vi "GET Async.vi"(0 "client handle":T1, 1 "output file":path=path "", 5 "url":string, 11 "error in (no error)":errorcluster, 12 "timeout (10000)":i32=10000) -> (4 "client handle out":T1, 6 "get async handle":T2, 10 "headers":string, 15 "error out":errorcluster)   [LabVIEW 2019, in "HTTP Client Extensions.lvlib" / "Get Async.lvlib"]
uses:
  Get Async.lvlib
  <vilib>/httpClient/ClientHandle.ctl
  controls/Refnum Type.ctl
  controls/Refnum Type - Enum.ctl
  HTTP GET Async/GET Async.lvclass
  <vilib>/httpClient/LabVIEWHTTPClient.lvlib
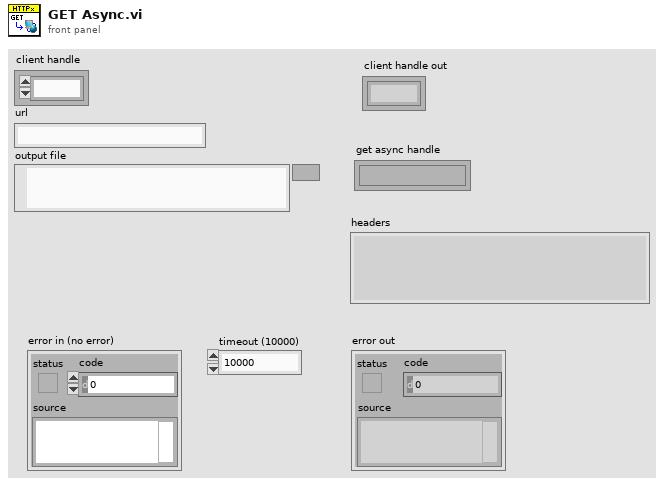
[diagram p1: front panel]
types:
  T1 = typedef "LabVIEWHTTPClient.lvlib/ClientHandle.ctl" = refnum<k1>
  T2 = typedef "HTTP Client Extensions.lvlib/Get Async.lvlib/Refnum Type.ctl" = refnum<k1>
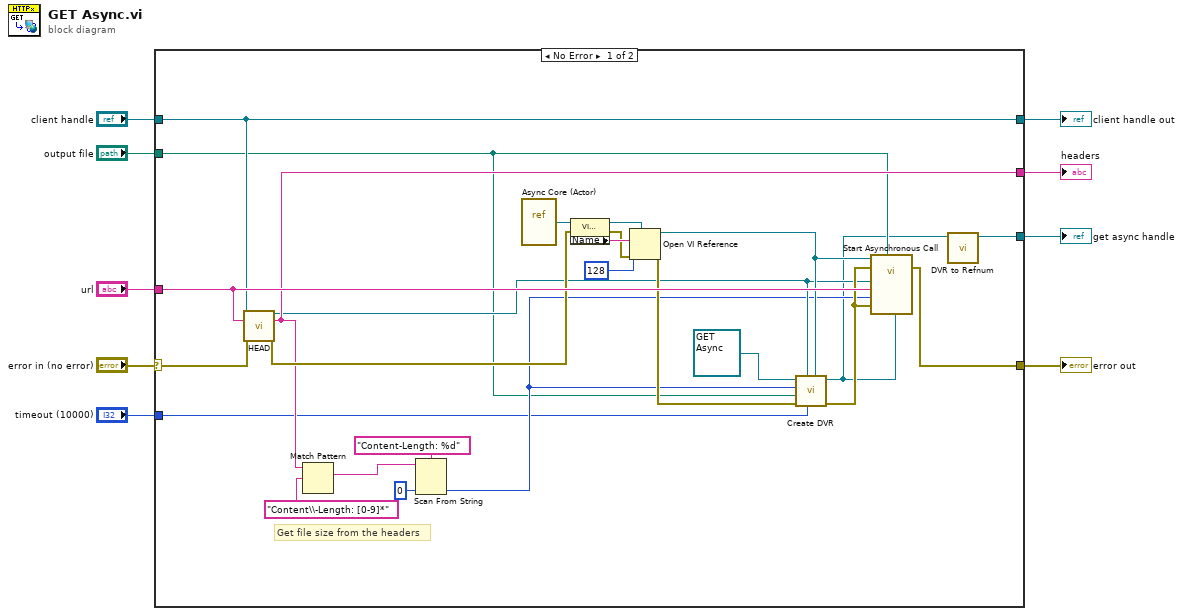
[diagram p0: block diagram]
diagram:
  n1 = case shown="No Error" "error in (no error)" {
    selector: "error in (no error)" -> [w34 w36]
    tunnel: "url" -> [w33 _]
    tunnel: [w24 w36] -> w7
    tunnel: [w11 _] -> w2
    tunnel: "output file" -> [w13 _]
    tunnel: "client handle" -> [w21 w35]
    tunnel: [w21 w35] -> w4
    tunnel: [w20 _] -> w3
    tunnel: "timeout (10000)" -> [w10 _]
    frame No Error {
      # "Get file size from the headers"
      n2 = call <vilib>:"HEAD.vi"("client handle"=w21, "url"=w33, "error in (no error)"=w34) -> ("client handle out"=w16:T1, "headers"=w20:string, "error out"=w22:errorcluster)  [unwired: 10 in]
      n3 = Match Pattern(string=w20, regular expression="Content\\-Length: [0-9]*") -> (match substring=w31:string)  [unwired: 1 in, 3 out]
      n4 = Scan From String(format string="Content-Length: %d", input string=w31, default 1=i64 0 ("default value 1")) -> (output 1=w14:i64)  [unwired: 2 in, 3 out]
      n5 = vi-ref "Async Core (Actor).vi"() -> (w28:refnum<vi>)
      n6 = property class="VI (strict)"(reference=w28, error in=w22) -> (reference out=w26:refnum<vi>, error out=w23:errorcluster, "Name"=w27:string)
      n7 = Open VI Reference(type specifier VI Refnum (for type only)=w26, vi path=w27, options=128, error in (no error)=w23) -> (vi reference=w17:refnum<vi>, error out=w18:errorcluster)  [unwired: 2 in]
      n8 = call "Create DVR.vi"("Actor Ref"=w17, "timeout (10000)"=w10, "client handle"=w16, "error in (no error)"=w18, "output file"=w13, "file size"=w14, "GET Async in"=refnum<class "GET Async.lvclass"> refnum) -> ("error out"=w19:errorcluster, "HTTP GET Async ref"=w12:refnum<data-value>)  [unwired: 3 in]
      n9 = call-by-ref "Start Asynchronous Call"(reference=w17, error in=w19, "HTTP GET Async ref"=w12, "output file"=w13, 8:"error in (no error)"=w19, "file size (bytes)"=w14, "file url"=w33, "client handle"=w16) -> (error out=w24:errorcluster)  [unwired: 6 in, 1 out]
      n10 = call "DVR to Refnum.vi"("Data Value Reference in"=w12) -> ("Refnum out"=w11:T2)  [unwired: 10 in]
    }
    frame Error {
    }
  }
  "error out" <- w7
  "get async handle" <- w2
  "client handle out" <- w4
  "headers" <- w3
